vi "oa_Auto Detect Decreasing RPM Step.vi"(0 "reset?":bool, 5 "speed(RPM)":dbl[](array[numeric]), 7 "start input":dbl, 9 "end input":dbl, 11 "step input":dbl) -> (4 "start output":dbl, 6 "end output":dbl, 8 "step output":dbl, 15 "step found?":bool)   [LabVIEW 2017]
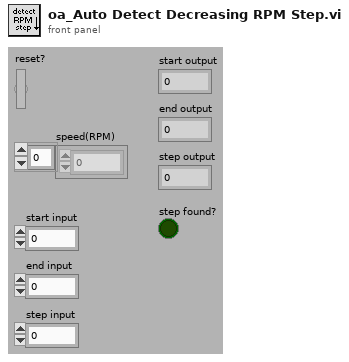
[diagram p1: front panel]
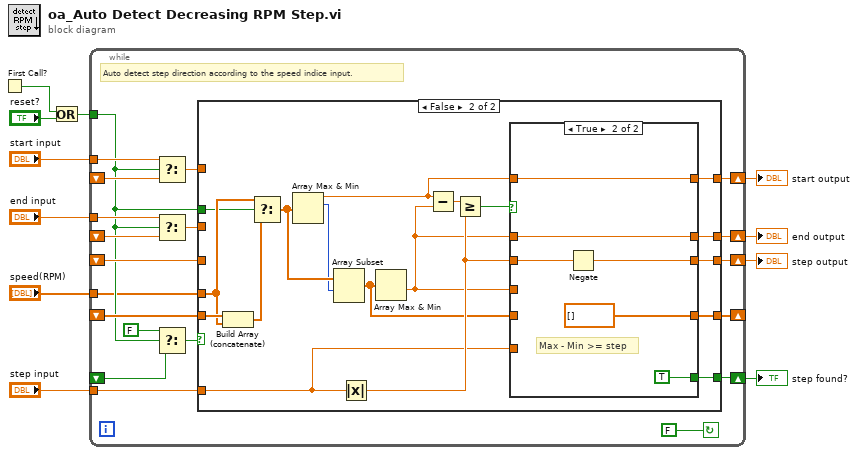
[diagram p0: block diagram]
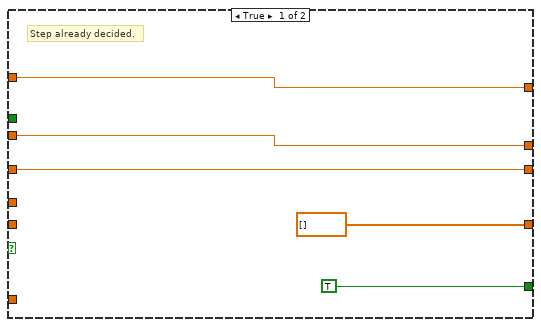
[diagram p2: hidden frame]
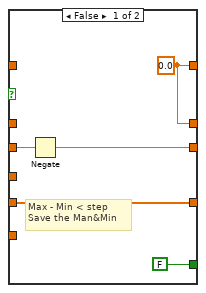
[diagram p3: hidden frame]
diagram:
  n1 = First Call?() -> (First Call?: T/F=w6:bool)
  n2 = Or(x=w6, y="reset?") -> (x .or. y?=w11:bool)
  n3 = while {
    tunnel: w11 -> [w13]
    tunnel: "speed(RPM)" -> [w12]
    shift-right: [w25] -> _
    shift-left: _ -> [w30]
    shift-right: [w24] -> w1
    shift-left: _ -> [w29]
    tunnel: "step input" -> [w27]
    shift-right: [w21] -> w2
    shift-left: _ -> [w20]
    shift-right: [w22] -> w3
    shift-left: _ -> [w16]
    shift-right: [w23] -> w4
    shift-left: _ -> [w19]
    tunnel: "start input" -> [w18]
    tunnel: "end input" -> [w15]
    stop <- FALSE continue-if-true
    # "Auto detect step direction according to the speed indice input."
    n4 = Select(t=w18, s=w13, f=w19) -> (s? t:f=w17:dbl)
    n5 = Select(t=w15, s=w13, f=w16) -> (s? t:f=w14:dbl)
    n6 = Select(t=FALSE, s=w13, f=w29) -> (s? t:f=w26:bool)
    n7 = case shown="False" w26 {
      tunnel: w30 -> [_ w54]
      tunnel: w12 -> [_ w53]
      tunnel: w13 -> [_ w48]
      tunnel: w27 -> [_ w41]
      tunnel: [dbl[] [] ("appended array") w47] -> w25
      tunnel: [TRUE w46] -> w24
      tunnel: [w34 w45] -> w23
      tunnel: [w33 w44] -> w22
      tunnel: [w32 w43] -> w21
      tunnel: w17 -> [w34 _]
      tunnel: w14 -> [w33 _]
      tunnel: w20 -> [w32 _]
      frame True {
        # "Step already decided."
      }
      frame False {
        n8 = Build Array (concatenate)(w54, w53) -> (w49:dbl[])
        n9 = Select(t=w53, s=w48, f=w49) -> (s? t:f=w40:dbl[])
        n10 = Array Max & Min(array=w40) -> (max value=w42:dbl, max index (indices)=w39:i32)  [unwired: 2 out]
        n11 = Array Subset(array=w40, index=w39) -> (w37:dbl[])  [unwired: 1 in]
        n12 = Absolute Value(x=w41) -> (abs(x)=w52:dbl)
        n13 = Array Max & Min(array=w37) -> (min value=w38:dbl)  [unwired: 3 out]
        n14 = Subtract(x=w42, y=w38) -> (x-y=w50:dbl)
        n15 = Greater Or Equal?(x=w50, y=w52) -> (x >= y?=w51:bool)
        n16 = case shown="True" w51 {
          tunnel: [w58 w63] -> w45
          tunnel: [w58 w62] -> w44
          tunnel: [w55 w60] -> w43
          tunnel: w52 -> [w56 w61]
          tunnel: [w57 dbl[] [] ("appended array")] -> w47
          tunnel: [FALSE TRUE] -> w46
          tunnel: w38 -> [_ _]
          tunnel: w42 -> [_ w63]
          tunnel: w41 -> [_ _]
          tunnel: w38 -> [_ w62]
          tunnel: w37 -> [w57 _]
          frame False {
            w58 = 0.0 ("t")
            # "Max - Min < step\nSave the Man&Min"
            n17 = Negate(x=w56) -> (-x=w55:dbl)
          }
          frame True {
            # "Max - Min >= step"
            n18 = Negate(x=w61) -> (-x=w60:dbl)
          }
        }
      }
    }
  }
  "start output" <- w4
  "end output" <- w3
  "step output" <- w2
  "step found?" <- w1
